vi "SetDebugData.vi"(2 "DebugData":T1, 5 "error in (no error)":errorcluster) -> (19 "error out":errorcluster)   [LabVIEW 2014, in "IndoorData.lvclass"]
uses:
  IndoorData.lvclass
  DebugData.ctl
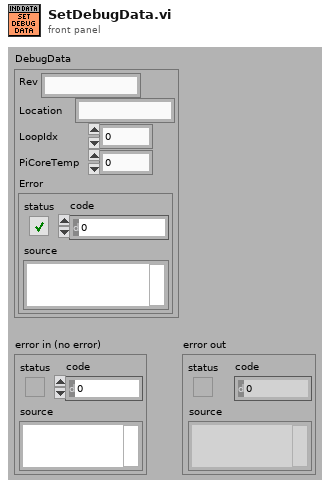
[diagram p1: front panel]
types:
  T1 = typedef "IndoorData.lvclass/DebugData.ctl" = cluster{"Rev":string, "Location":string, "LoopIdx":i32, "PiCoreTemp":dbl, "Error":errorcluster}
  T2 = typedef "IndoorData.lvclass/ObjectAttributes.ctl" = cluster{"DebugData":T1, "Actual":T3}
  T3 = typedef "IndoorData.lvclass/ActualValues.ctl" = cluster{"Time":dbl, "Temp":dbl, "RH":dbl}
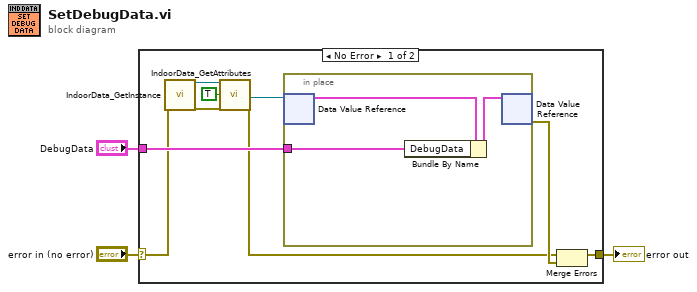
[diagram p0: block diagram]
diagram:
  n1 = case shown="No Error" "error in (no error)" {
    selector: "error in (no error)" -> [w6 w16]
    tunnel: [w10 w16] -> w2
    tunnel: "DebugData" -> [w12 _]
    frame No Error {
      n2 = call "IndoorData_GetInstance.vi"("error in (no error)"=w6) -> ("reference out"=w7:refnum<class "IndoorData.lvclass">, "error out"=w8:errorcluster)  [unwired: 14 in, 3 out]
      n3 = call "IndoorData_GetAttributes.vi"("reference in"=w7, "OnlyGetDvrReference(False)"=TRUE, "error in (no error)"=w8) -> ("DataRef"=w5:refnum<data-value>, "error out"=w9:errorcluster)  [unwired: 13 in, 2 out]
      n4 = in-place {
        in-place-border: w12 -> [w15]
        n5 = in-place-dvr #1(w5) -> (w14:T2)  [unwired: 1 out]
        n6 = Bundle By Name(cluster=w14, "DebugData"=w15) -> (w13:T2)
        n7 = in-place-dvr #1(w13) -> (w11:errorcluster)  [unwired: 1 out]
      }
      n8 = Merge Errors(w9, w11) -> (w10:errorcluster)
    }
    frame Error {
    }
  }
  "error out" <- w2
